vi "Swap Neighborhood.vi"(11 "Schedule In":u16[](array[numeric])) -> (3 "Schedule Out":u16[](array[numeric]))   [LabVIEW 2013]
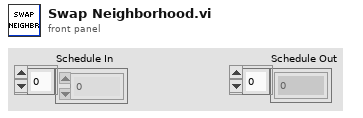
[diagram p1: front panel]
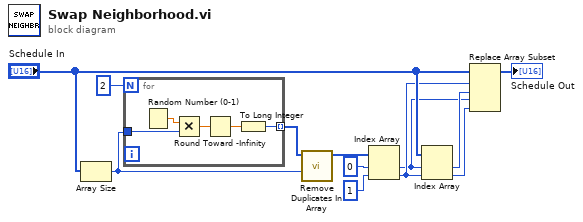
[diagram p0: block diagram]
diagram:
  n1 = Array Size(array="Schedule In") -> (size(s)=w8:i32)
  n2 = for {
    N: 2 -> [_]
    tunnel: w8 -> [w16]
    tunnel: [w13] -> w9 mode=indexing
    n3 = Random Number (0-1)() -> (number: 0 to 1=w17:dbl)
    n4 = Multiply(x=w17, y=w16) -> (x*y=w15:dbl)
    n5 = Round Toward -Infinity(1:w15) -> (0:w14:dbl)
    n6 = To Long Integer(number=w14) -> (32bit integer=w13:i32)
  }
  n7 = call "Remove Duplicates In Array.vi"("Max Index Bound"=w8, "Random Numbers Array"=w9) -> ("Random Numbers Array without Duplicates"=w7:i32[])  [unwired: 9 in]
  n8 = Index Array(array=w7, index #1=0 ("index"), index #2=1 ("index")) -> (element #1=w2:i32, element #2=w4:i32)
  n9 = Index Array(array="Schedule In", index #1=w2, index #2=w4) -> (element #1=w3:u16, element #2=w1:u16)
  n10 = Replace Array Subset(array="Schedule In", new element #1=w3, index #1=w4, new element #2=w1, index #2=w2) -> (→"Schedule Out":u16[])
